vi "macro_Translation2d_X_Y.vi"   [LabVIEW 2019, in "Trajectory_Library.lvlib"]
uses:
  Trajectory_Library.lvlib
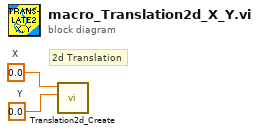
[diagram p0: block diagram]
diagram:
  w1 = 0.0  # X
  w2 = 0.0  # Y
  # "2d Translation"
  n1 = call "Translation2d_Create.vi"("Y"=w2, "X"=w1) -> ()  [unwired: 9 in, 1 out]
